vi "convert_I16-to-DACvalue.vi"(10 "DAC Value (I16)":u16) -> (2 "DAC value (sgl)":sgl)   [LabVIEW 2013]
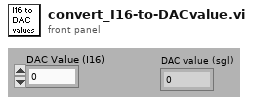
[diagram p1: front panel]
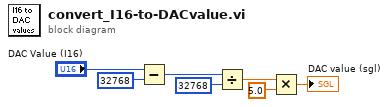
[diagram p0: block diagram]
diagram:
  n1 = Subtract(x="DAC Value (I16)", y=u16 32768) -> (x-y=w5:i32)
  n2 = Divide(x=w5, y=32768) -> (x/y=w3:dbl)
  n3 = Multiply(x=w3, y=5.0 ("DACS Range")) -> (x*y=→"DAC value (sgl)":dbl)
